vi "Tree_Filter_1 Text Filter.vi"(7 "Filter On":enum16{"Left Cell String", "Child Tag"}(ring), 10 "Filter":string, 11 "Tree Array in":T1(array[cluster])) -> (2 "Keep?":bool[](array[boolean]), 3 "Tree Array out":T1(array[cluster]))   [LabVIEW 2023]
doc: "Basic tree text filter works on left cell string or tag. The tree array out is the same as the arrray in. This must go through part 2, to mainting the tree heirarchy. The output boolean array indicates retained (filter pass) items."
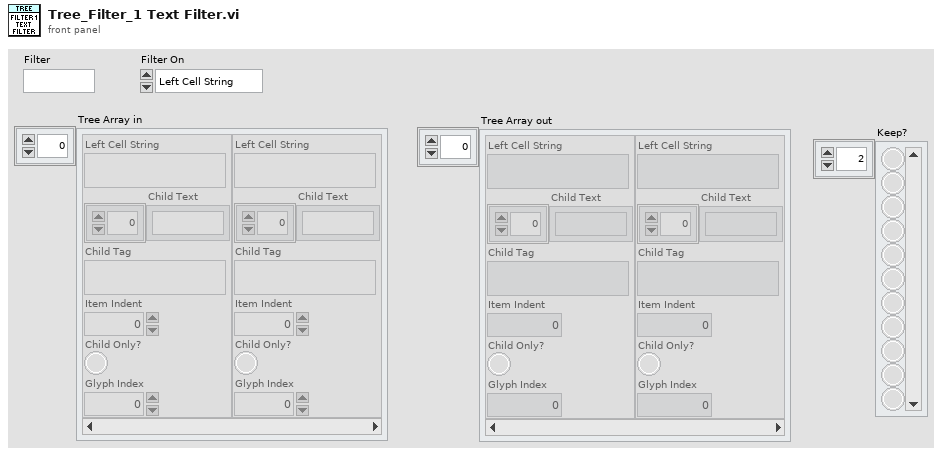
[diagram p1: front panel]
types:
  T1 = cluster{"Left Cell String":string, "Child Text":string[], "Child Tag":string, "Item Indent":i32, "Child Only?":bool, "Glyph Index":i32}[]
  T2 = enum16{"Unknown", "Base", "Scripting", "Private", "Deprecated", "None", "Divider"}
  T3 = cluster{"Index":u16, "Property Type":enum16{"Unknown", "Base", "Scripting", "Private", "Deprecated", "None", "Divider"}, "ID String":string, "Dotted ID String":string, "Class":string, "Parent":string, "Display name full":string, "Display name short":string, "Parents Array":string[], "Indent":u16}
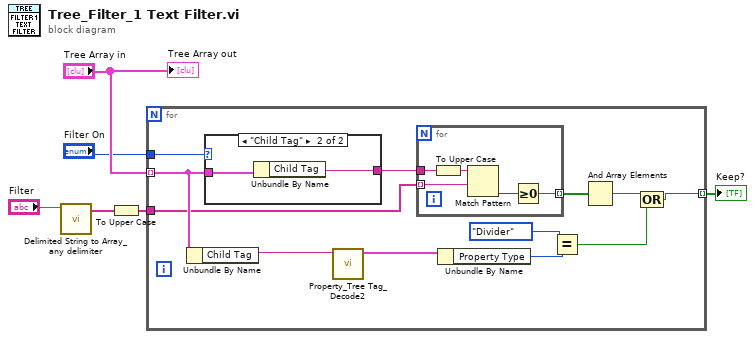
[diagram p0: block diagram]
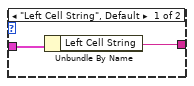
[diagram p2: hidden frame]
diagram:
  n1 = call "Delimited String to Array_any delimiter.vi"("Delimted String"="Filter") -> ("Array"=w1:string[])  [unwired: 10 in]
  n2 = To Upper Case(1:w1) -> (0:w3:string[])
  n3 = for {
    tunnel: "Tree Array in" -> [w16] mode=indexing
    tunnel: w3 -> [w9]
    tunnel: [w10] -> w6 mode=indexing
    tunnel: "Filter On" -> [w17]
    n4 = Unbundle By Name(w16) -> ("Child Tag"=w15:string)
    n5 = case shown="\"Child Tag\"" w17 {
      tunnel: w16 -> [w25 w27]
      tunnel: [w24 w26] -> w18
      frame "Left Cell String", Default {
        n6 = Unbundle By Name(w25) -> ("Left Cell String"=w24:string)
      }
      frame "Child Tag" {
        n7 = Unbundle By Name(w27) -> ("Child Tag"=w26:string)
      }
    }
    n8 = call "Property_Tree Tag_Decode2.vi"("Tag In"=w15) -> ("TagData"=w14:T3)  [unwired: 10 in]
    n9 = for {
      tunnel: w18 -> [w23]
      tunnel: w9 -> [w22] mode=indexing
      tunnel: [w19] -> w8 mode=indexing
      n10 = To Upper Case(1:w23) -> (0:w20:string)
      n11 = Match Pattern(string=w20, regular expression=w22) -> (offset past match=w21:i32)  [unwired: 1 in, 3 out]
      n12 = Greater Or Equal To 0?(x=w21) -> (x >= 0?=w19:bool)
    }
    n13 = Unbundle By Name(w14) -> ("Property Type"=w12:T2)
    n14 = Equal?(x=T2."Divider" ("Property Type"), y=w12) -> (x = y?=w11:bool)
    n15 = And Array Elements(Boolean array=w8) -> (logical AND=w7:bool)
    n16 = Compound Arithmetic op=OR(w7, w11) -> (w10:bool)
  }
  "Keep?" <- w6
  "Tree Array out" <- "Tree Array in"
